vi "leybold QMH.vi"() -> ()   [LabVIEW 2023]
uses:
  usr/local/natinst/LabVIEW-2023-64/examples/Design Patterns/Queued Message Handler/support/QMH Fundamentals - Message Cluster.ctl
  <vilib>/Instr/_visa.llb/VISA Configure Serial Port (Instr).vi
  <vilib>/Utility/error.llb/Error Cluster From Error Code.vi
  <vilib>/ErrorRing/Error Ring.xnode
panel:
  in  "Stop":bool
  in  "recipes":bool
  in  "Tab Control":enum32{"Control", "Vacuum", "Metals", "Oxides"}(tab)
  out "REF Power (W)":i16
  in  "FWD Power (W)":bool=TRUE
  in  "CL":bool
  in  "CT":bool
  in  "RF Source":bool
  out "PFG600":string
  out "read buffer":string
  in  "+100":bool
  out "DC Bias (V)":i16
  in  "Ar (SCCM)":bool
  in  "O2 (SCCM)":bool
  in  "Gas":bool
  in  "+10":bool
  in  "+1":bool
  in  "-1":bool
  in  "-10":bool
  in  "-100":bool
  in  "GAS Boost":bool
  in  "Timer":bool
  in  "Matchbox mode":bool
  in  "TimerOn":bool
  out "PR4000":string
  in  "P1":bool
  in  "P2":bool
  in  "P3":bool
  out "Timer end":timestamp format="%<%H:%M:%S>T"
  out "Time":timestamp format="%<%H:%M:%S\n%x>T"
  in  "RS232":bool
  out "Waveform Chart":waveform(dbl)(graph)
  in  "1h":bool
  in  "8h":bool
  in  "24h":bool
  in  "All":bool
  out "Pressure (mbar)":dbl format="%#_6e"
  # "GENERATOR"
  # "MFC"
  # "TIMER"
  # "PRESETS"
  # "DEBUG"
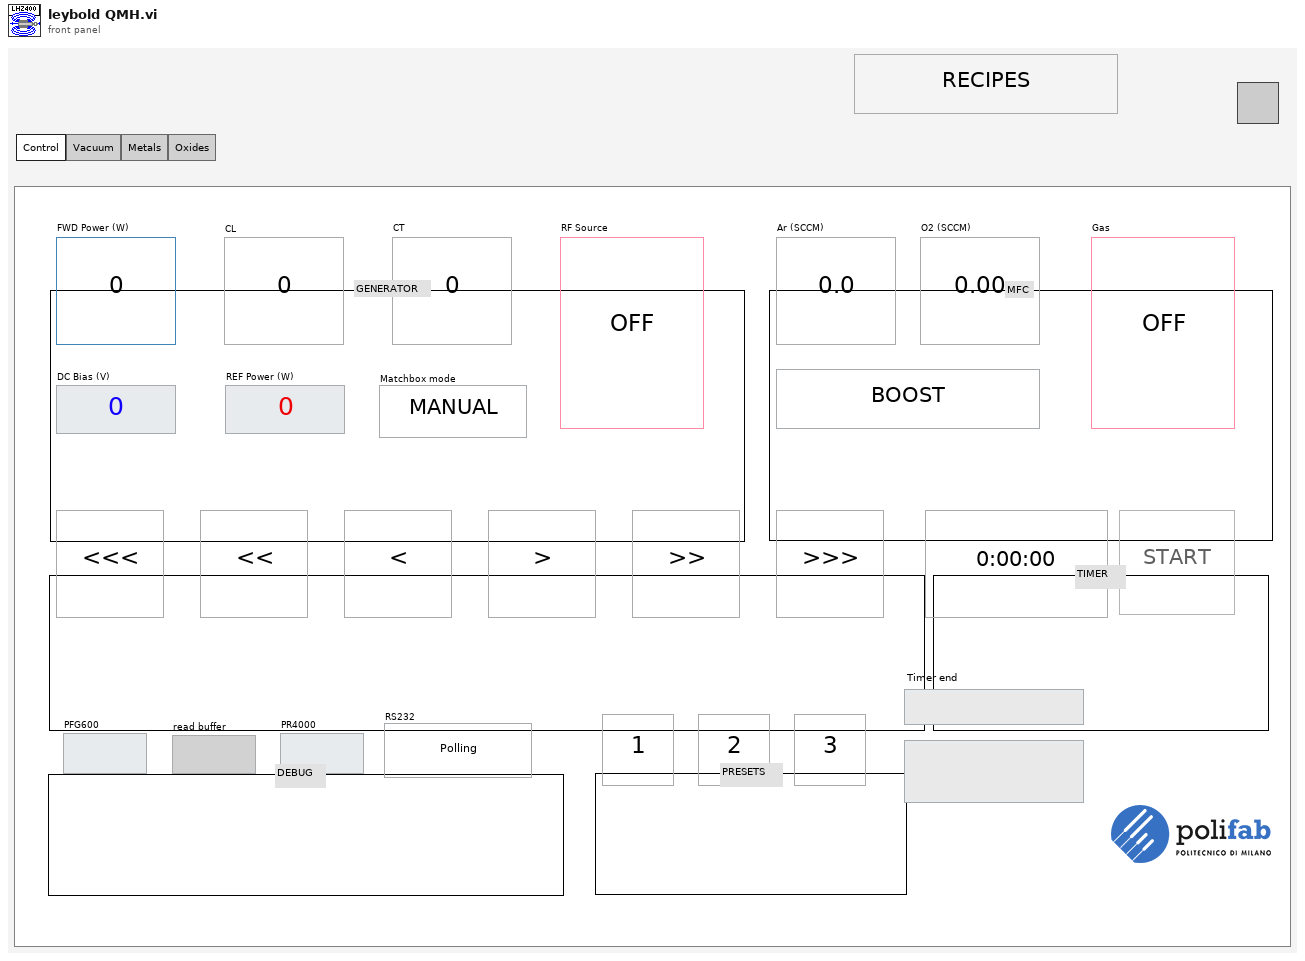
[diagram p1: front panel]
types:
  T1 = typedef "QMH Fundamentals - Message Cluster.ctl" = cluster{"Message":string, "Message Data":variant}
  T2 = cluster{"Message":string, enum16{"FWD", "CL", "CT", "Ar", "O2", "Timer"}}
  T3 = enum8{"Enabled", "Disabled", "Disabled and Grayed Out"}
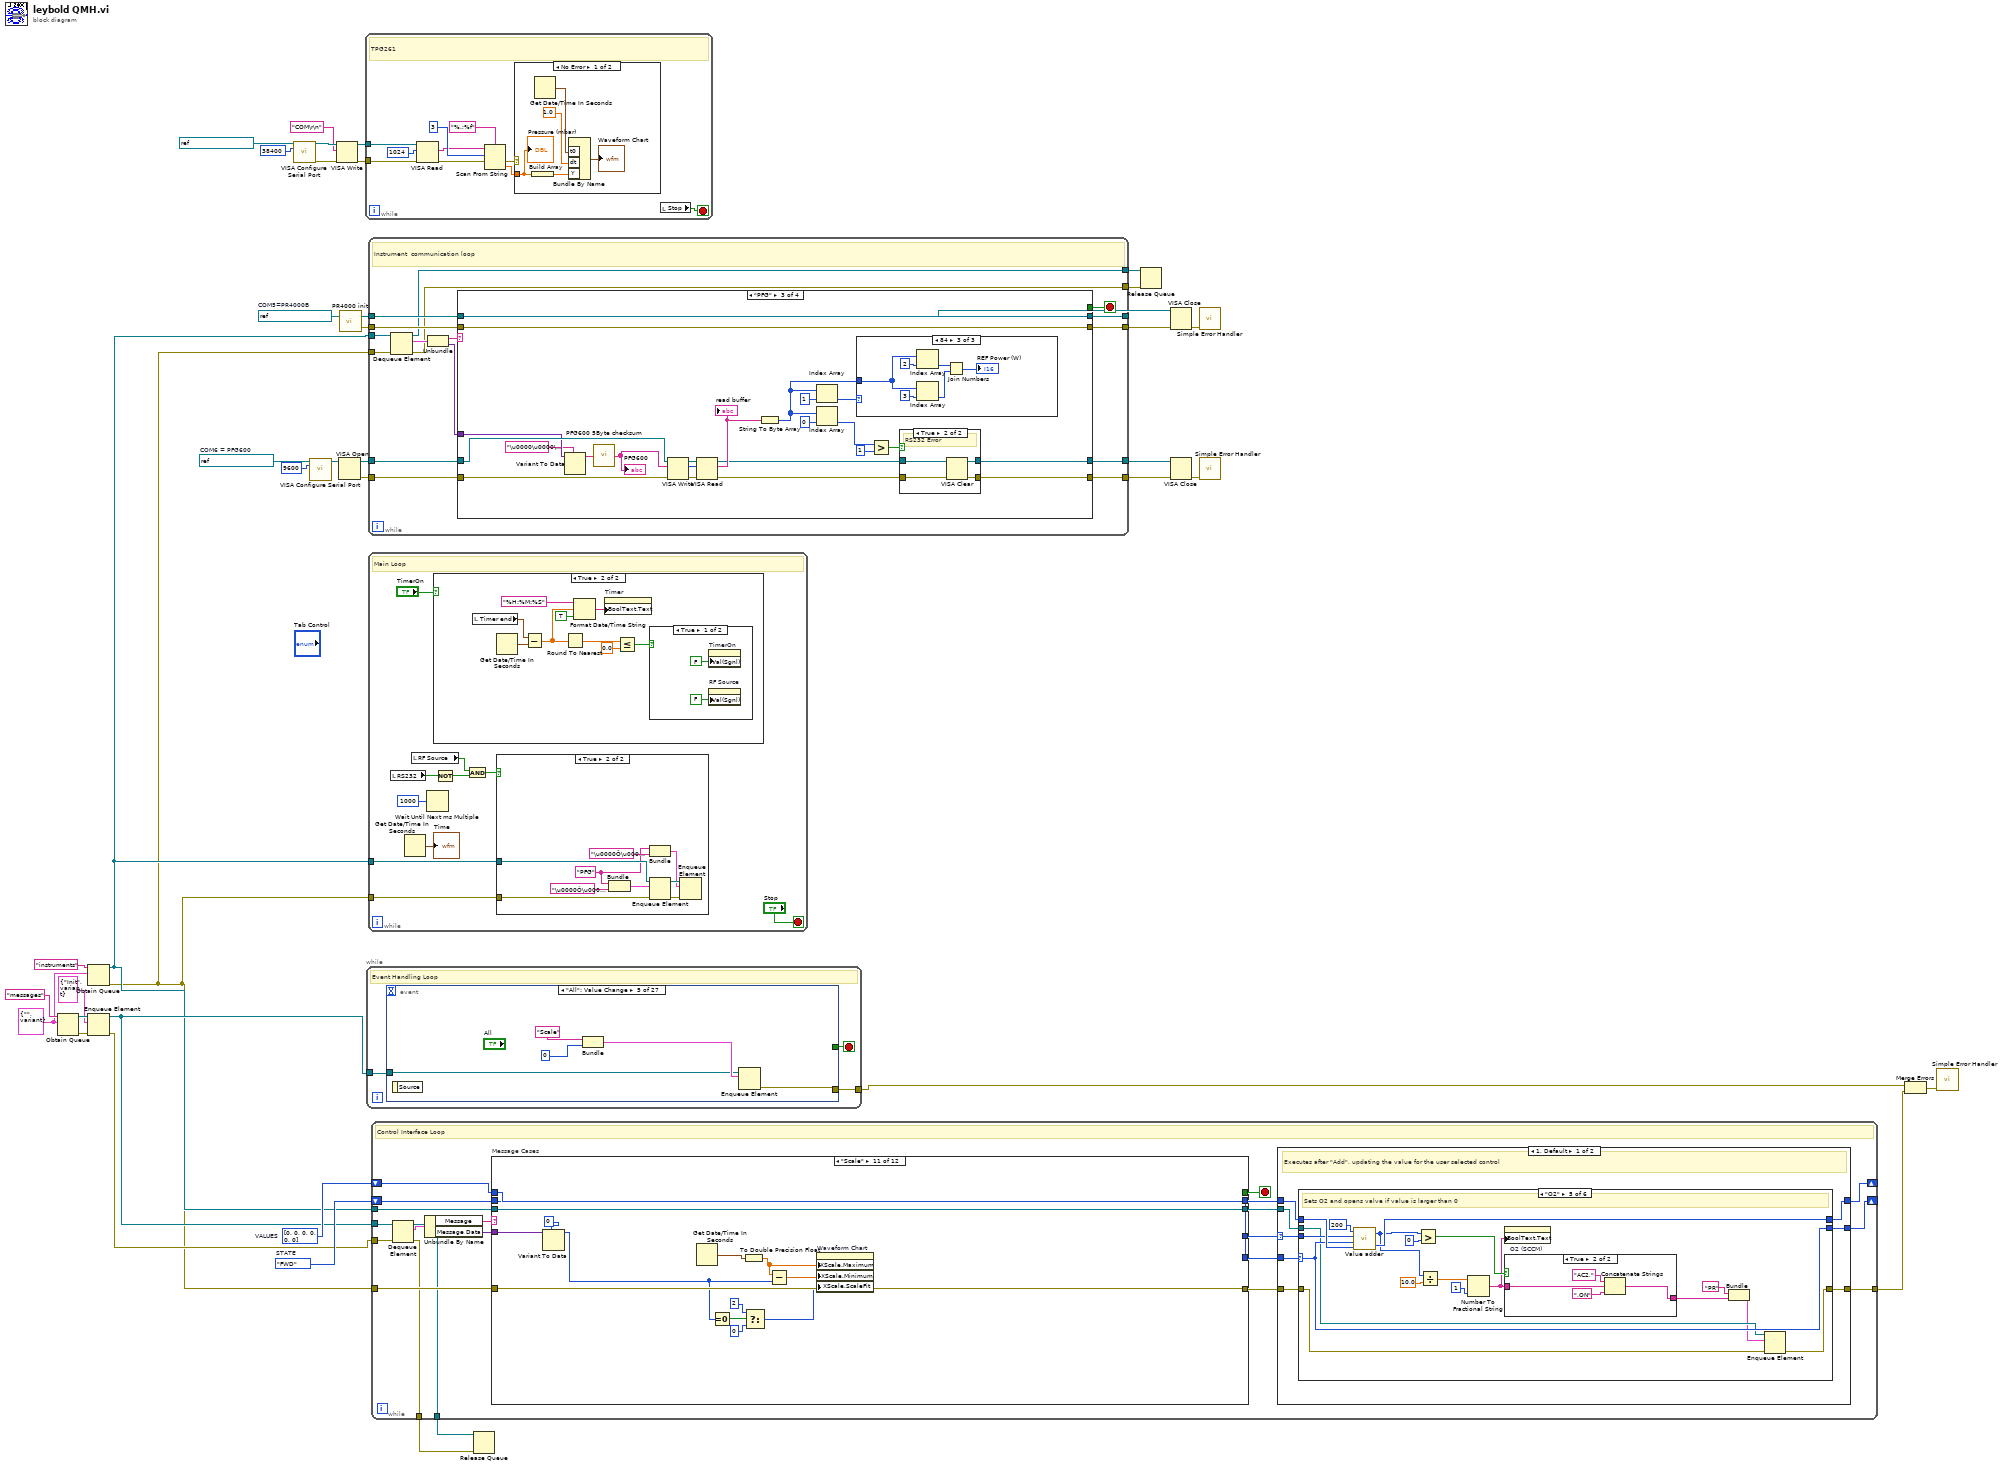
[diagram p0: block diagram]
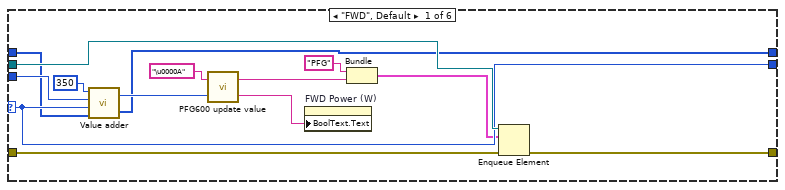
[diagram p2: hidden frame]
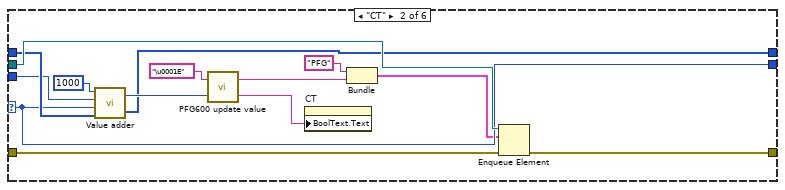
[diagram p3: hidden frame]
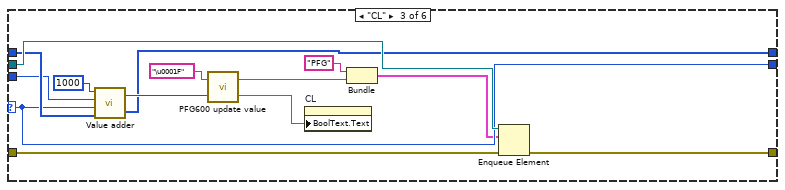
[diagram p4: hidden frame]
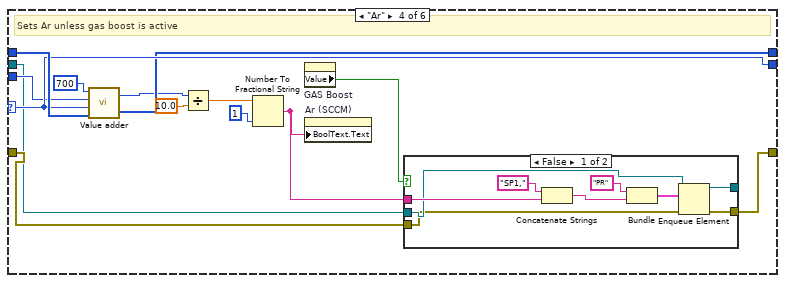
[diagram p5: hidden frame]
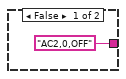
[diagram p7: hidden frame]
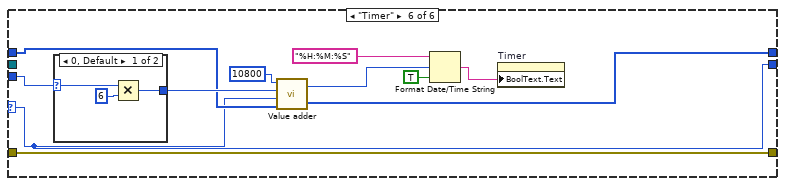
[diagram p8: hidden frame]
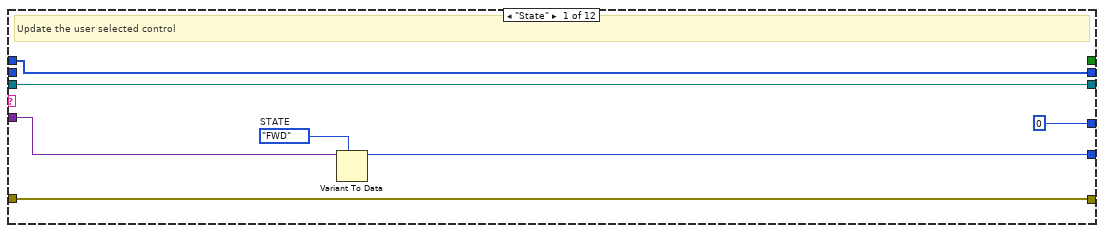
[diagram p11: hidden frame]
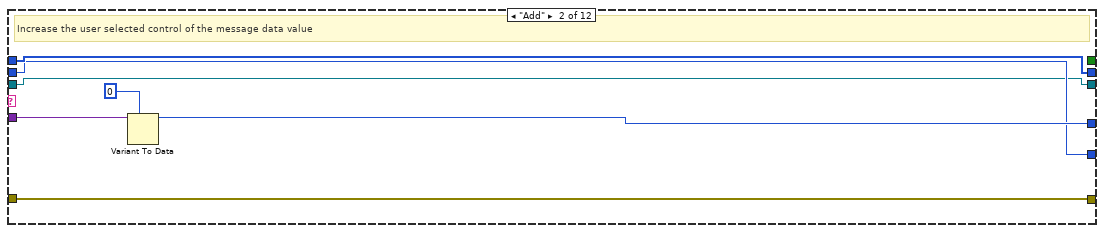
[diagram p12: hidden frame]
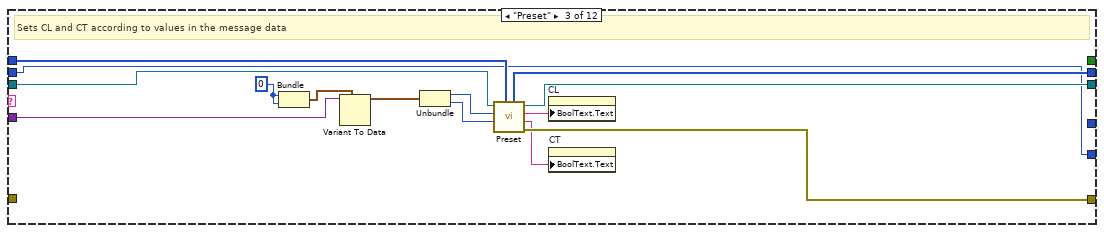
[diagram p13: hidden frame]
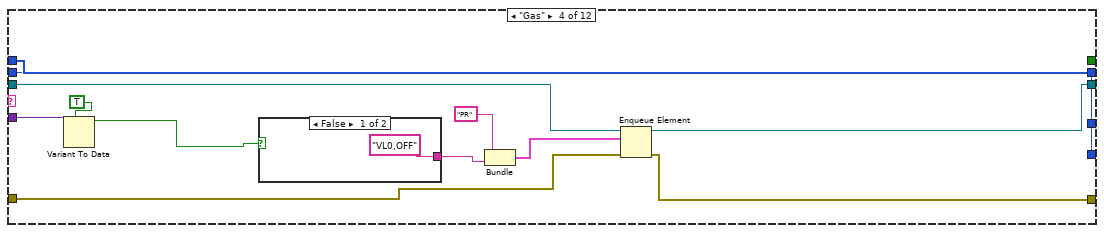
[diagram p14: hidden frame]
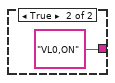
[diagram p15: hidden frame]
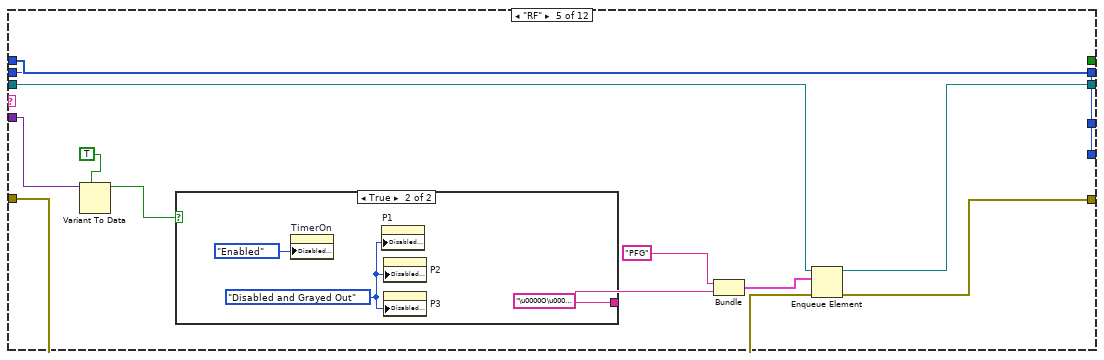
[diagram p16: hidden frame]
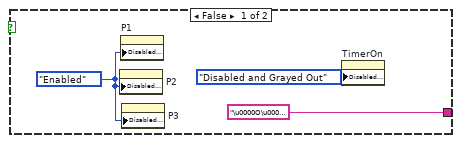
[diagram p17: hidden frame]
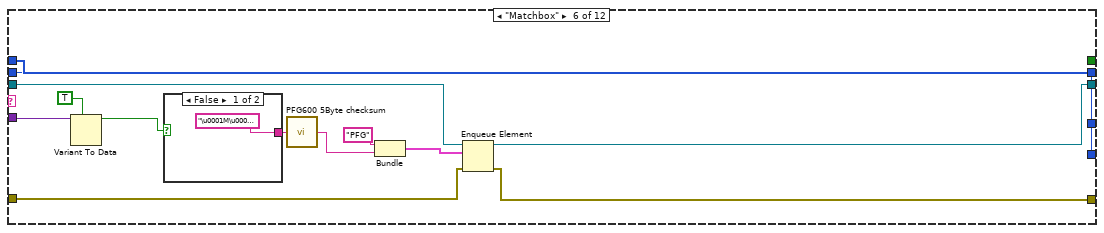
[diagram p18: hidden frame]
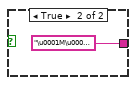
[diagram p19: hidden frame]
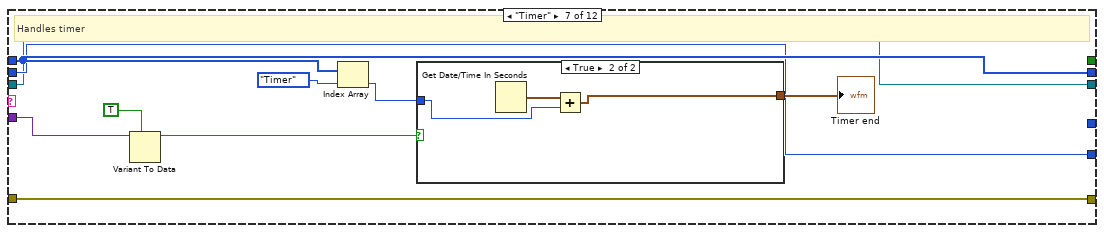
[diagram p20: hidden frame]
diagram:
  w20 = i16[] [0, 0, 0, 0, 0, 0]  # VALUES
  w21 = enum16{"FWD", "CL", "CT", "Ar", "O2", "Timer"}."FWD"  # STATE
  w11 = T1 {"Message"="", "Message Data"=variant} ("Message Cluster")
  w34 = refnum<visa-resource-name> "ASRL33::INSTR"  # COM5=PR4000B
  w5 = refnum<visa-resource-name> "ASRL34::INSTR"  # COM6 = PFG600
  n1 = Obtain Queue(name (unnamed)="messages", element data type=w11) -> (queue out=w25:refnum<queue>, error out=w26:errorcluster)  [unwired: 3 in, 1 out]
  n2 = Obtain Queue(name (unnamed)="instruments", element data type=w11) -> (queue out=w10:refnum<queue>, error out=w9:errorcluster)  [unwired: 3 in, 1 out]
  n3 = Enqueue Element(queue=w25, element=T1 {"Message"="Init", "Message Data"=variant}, error in (no error)=w26) -> (queue out=w19:refnum<queue>, error out=w14:errorcluster)  [unwired: 1 in, 1 out]
  n4 = call-poly "VISA Configure Serial Port"("VISA resource name"=refnum<visa-resource-name> "ASRL36::INSTR", "baud rate (9600)"=u32 38400) -> ("VISA resource name out"=w29:refnum<visa-resource-name>, "error out"=w30:errorcluster)  [unwired: 12 in]
  n5 = call-poly "VISA Configure Serial Port"("VISA resource name"=w5, "baud rate (9600)"=u32 9600) -> ("VISA resource name out"=w6:refnum<visa-resource-name>)  [unwired: 12 in, 1 out]
  n6 = VISA Write(VISA resource name=w29, write buffer="COM\r\n", error in (no error)=w30) -> (VISA resource name out=w31:refnum<visa-resource-name>, error out=w27:errorcluster)  [unwired: 1 out]
  n7 = VISA Open(VISA resource name=w6) -> (VISA resource name=w39:refnum<visa-resource-name>, error out=w40:errorcluster)  [unwired: 4 in]
  n8 = call "PR4000 init.vi"("VISA Refnum in"=w34) -> ("error out"=w17:errorcluster, "VISA Refnum out"=w18:refnum<visa-resource-name>)  [unwired: 1 in]
  n9 = while {
    tunnel: w31 -> [w50]
    tunnel: w27 -> [w49]
    stop <- w41 stop-if-true
    # "TPG261"
    n10 = VISA Read(VISA resource name=w50, byte count=u32 1024, error in (no error)=w49) -> (read buffer=w45:string, error out=w43:errorcluster)  [unwired: 2 out]
    n11 = Scan From String(format string="%.;%f" ("Format-String"), input string=w45, initial scan location=u32 3 ("offset (0)"), error in=w43) -> (error out=w42:errorcluster, output 1=w44:dbl)  [unwired: 1 in, 2 out]
    n12 = case shown="No Error" w42 {
      tunnel: w44 -> [w52 _]
      frame No Error {
        n13 = Build Array(w52) -> (w55:dbl[])
        n14 = Get Date/Time In Seconds() -> (seconds since 1Jan1904=w51:timestamp)
        n15 = Bundle By Name("t0"=w51, "dt"=1.0, "Y"=w55) -> (→"Waveform Chart":waveform(dbl))  [unwired: 1 in]
        "Pressure (mbar)" <- w52
      }
      frame Error {
      }
    }
    n16 = local read "Stop"() -> (w41:bool)
  }
  n17 = while {
    tunnel: w19 -> [w58]
    tunnel: [w56] -> w23
    stop <- w57 stop-if-true
    # "Event Handling Loop"
    n18 = event shown="[4] \"All\": Value Change" {
      selector: _ -> [_ _ _ _ _ _ _ _ _ _ _ _ _ _ _ _ _ _ _ _ _ _ _ _ _ _ _]
      dyn-events: _ -> [_ _ _ _ _ _ _ _ _ _ _ _ _ _ _ _ _ _ _ _ _ _ _ _ _ _ _]
      timeout: _ -> [_ _ _ _ _ _ _ _ _ _ _ _ _ _ _ _ _ _ _ _ _ _ _ _ _ _ _]
      tunnel: [TRUE _ _ _ _ _ _ _ _ _ _ _ _ _ _ _ _ _ _ _ _ _ _ _ _ _ _] -> w57
      tunnel: w58 -> [w62 w64 w69 w74 w79 w83 w89 w93 w97 w101 w105 w109 w112 w115 w118 w121 w124 w129 w134 _ w142 w145 w152 w158 w164 w169 _]
      tunnel: [w61 w63 w68 w73 w78 _ _ _ _ _ _ w108 w111 w114 w117 w120 w123 w128 w133 _ _ _ _ _ _ w168 _] -> w56
      event "Stop": Value Change {
        # "Stop the VI."
        # "Enqueue an \"Exit\" message. Note that the Enqueue Element At Opposite End function is used to place this priority \"Exit\" message at the front of the queue ahead of all other messages."
        n19 = event-data() -> ()  [unwired: 1 in, 1 out]
        n20 = Enqueue Element At Opposite End(queue=w62, element=T1 {"Message"="Exit", "Message Data"=variant}) -> (error out=w61:errorcluster)  [unwired: 2 in, 2 out]
      }
      event "1h": Value Change {
        n21 = event-data() -> ()  [unwired: 1 in, 1 out]
        n22 = Bundle("Scale", 3600) -> (w66:cluster{string, i32})  [unwired: 1 in]
        n23 = Enqueue Element(queue=w64, element=w66) -> (error out=w63:errorcluster)  [unwired: 2 in, 2 out]
      }
      event "8h": Value Change {
        n24 = event-data() -> ()  [unwired: 1 in, 1 out]
        n25 = Bundle("Scale", 28800) -> (w71:cluster{string, i32})  [unwired: 1 in]
        n26 = Enqueue Element(queue=w69, element=w71) -> (error out=w68:errorcluster)  [unwired: 2 in, 2 out]
      }
      event "24h": Value Change {
        n27 = event-data() -> ()  [unwired: 1 in, 1 out]
        n28 = Bundle("Scale", 86400) -> (w76:cluster{string, i32})  [unwired: 1 in]
        n29 = Enqueue Element(queue=w74, element=w76) -> (error out=w73:errorcluster)  [unwired: 2 in, 2 out]
      }
      event "All": Value Change {
        n30 = event-data() -> ()  [unwired: 1 in, 1 out]
        n31 = Bundle("Scale", 0) -> (w81:cluster{string, i32})  [unwired: 1 in]
        n32 = Enqueue Element(queue=w79, element=w81) -> (error out=w78:errorcluster)  [unwired: 2 in, 2 out]
      }
      event "CL": Value Change {
        w86 = FALSE ("FWD Power (W)")
        n33 = event-data() -> ()  [unwired: 1 in, 1 out]
        n34 = Enqueue Element(queue=w83, element=T2 {"Message"="State", enum."CL"}) -> ()  [unwired: 2 in, 3 out]
        n35 = property on="CT" class="Bool (strict)"("Value"=w86) -> ()  [unwired: 2 in, 2 out]
        n36 = property on="Timer" class="Bool (strict)"("Value"=w86) -> ()  [unwired: 2 in, 2 out]
        n37 = property on="CL" class="Bool (strict)"("Value"=TRUE ("CL")) -> ()  [unwired: 2 in, 2 out]
        n38 = property on="Ar (SCCM)" class="Bool (strict)"("Value"=w86) -> ()  [unwired: 2 in, 2 out]
        n39 = property on="O2 (SCCM)" class="Bool (strict)"("Value"=w86) -> ()  [unwired: 2 in, 2 out]
        n40 = property on="FWD Power (W)" class="Bool (strict)"("Value"=w86) -> ()  [unwired: 2 in, 2 out]
      }
      event "CT": Value Change {
        w88 = FALSE ("FWD Power (W)")
        n41 = event-data() -> ()  [unwired: 1 in, 1 out]
        n42 = Enqueue Element(queue=w89, element=T2 {"Message"="State", enum."CT"}) -> ()  [unwired: 2 in, 3 out]
        n43 = property on="CT" class="Bool (strict)"("Value"=TRUE ("CL")) -> ()  [unwired: 2 in, 2 out]
        n44 = property on="CL" class="Bool (strict)"("Value"=w88) -> ()  [unwired: 2 in, 2 out]
        n45 = property on="Timer" class="Bool (strict)"("Value"=w88) -> ()  [unwired: 2 in, 2 out]
        n46 = property on="Ar (SCCM)" class="Bool (strict)"("Value"=w88) -> ()  [unwired: 2 in, 2 out]
        n47 = property on="O2 (SCCM)" class="Bool (strict)"("Value"=w88) -> ()  [unwired: 2 in, 2 out]
        n48 = property on="FWD Power (W)" class="Bool (strict)"("Value"=w88) -> ()  [unwired: 2 in, 2 out]
      }
      event "Ar (SCCM)": Value Change {
        w92 = FALSE ("FWD Power (W)")
        n49 = event-data() -> ()  [unwired: 1 in, 1 out]
        n50 = Enqueue Element(queue=w93, element=T2 {"Message"="State", enum."Ar"}) -> ()  [unwired: 2 in, 3 out]
        n51 = property on="CL" class="Bool (strict)"("Value"=w92) -> ()  [unwired: 2 in, 2 out]
        n52 = property on="Ar (SCCM)" class="Bool (strict)"("Value"=TRUE ("CL")) -> ()  [unwired: 2 in, 2 out]
        n53 = property on="Timer" class="Bool (strict)"("Value"=w92) -> ()  [unwired: 2 in, 2 out]
        n54 = property on="CT" class="Bool (strict)"("Value"=w92) -> ()  [unwired: 2 in, 2 out]
        n55 = property on="O2 (SCCM)" class="Bool (strict)"("Value"=w92) -> ()  [unwired: 2 in, 2 out]
        n56 = property on="FWD Power (W)" class="Bool (strict)"("Value"=w92) -> ()  [unwired: 2 in, 2 out]
      }
      event "O2 (SCCM)": Value Change {
        w96 = FALSE ("FWD Power (W)")
        n57 = event-data() -> ()  [unwired: 1 in, 1 out]
        n58 = Enqueue Element(queue=w97, element=T2 {"Message"="State", enum."O2"}) -> ()  [unwired: 2 in, 3 out]
        n59 = property on="CL" class="Bool (strict)"("Value"=w96) -> ()  [unwired: 2 in, 2 out]
        n60 = property on="O2 (SCCM)" class="Bool (strict)"("Value"=TRUE ("CL")) -> ()  [unwired: 2 in, 2 out]
        n61 = property on="Timer" class="Bool (strict)"("Value"=w96) -> ()  [unwired: 2 in, 2 out]
        n62 = property on="CT" class="Bool (strict)"("Value"=w96) -> ()  [unwired: 2 in, 2 out]
        n63 = property on="Ar (SCCM)" class="Bool (strict)"("Value"=w96) -> ()  [unwired: 2 in, 2 out]
        n64 = property on="FWD Power (W)" class="Bool (strict)"("Value"=w96) -> ()  [unwired: 2 in, 2 out]
      }
      event "FWD Power (W)": Value Change {
        w100 = FALSE ("FWD Power (W)")
        n65 = event-data() -> ()  [unwired: 1 in, 1 out]
        n66 = Enqueue Element(queue=w101, element=T2 {"Message"="State", enum."FWD"}) -> ()  [unwired: 2 in, 3 out]
        n67 = property on="FWD Power (W)" class="Bool (strict)"("Value"=TRUE ("CL")) -> ()  [unwired: 2 in, 2 out]
        n68 = property on="O2 (SCCM)" class="Bool (strict)"("Value"=w100) -> ()  [unwired: 2 in, 2 out]
        n69 = property on="Timer" class="Bool (strict)"("Value"=w100) -> ()  [unwired: 2 in, 2 out]
        n70 = property on="CL" class="Bool (strict)"("Value"=w100) -> ()  [unwired: 2 in, 2 out]
        n71 = property on="Ar (SCCM)" class="Bool (strict)"("Value"=w100) -> ()  [unwired: 2 in, 2 out]
        n72 = property on="CT" class="Bool (strict)"("Value"=w100) -> ()  [unwired: 2 in, 2 out]
      }
      event "Timer": Value Change {
        w103 = FALSE ("FWD Power (W)")
        n73 = event-data() -> ()  [unwired: 1 in, 1 out]
        n74 = Enqueue Element(queue=w105, element=T2 {"Message"="State", enum."Timer"}) -> ()  [unwired: 2 in, 3 out]
        n75 = property on="CT" class="Bool (strict)"("Value"=w103) -> ()  [unwired: 2 in, 2 out]
        n76 = property on="Timer" class="Bool (strict)"("Value"=TRUE ("CL")) -> ()  [unwired: 2 in, 2 out]
        n77 = property on="CL" class="Bool (strict)"("Value"=w103) -> ()  [unwired: 2 in, 2 out]
        n78 = property on="Ar (SCCM)" class="Bool (strict)"("Value"=w103) -> ()  [unwired: 2 in, 2 out]
        n79 = property on="O2 (SCCM)" class="Bool (strict)"("Value"=w103) -> ()  [unwired: 2 in, 2 out]
        n80 = property on="FWD Power (W)" class="Bool (strict)"("Value"=w103) -> ()  [unwired: 2 in, 2 out]
      }
      event "-100": Value Change {
        n81 = event-data() -> ()  [unwired: 1 in, 1 out]
        n82 = Enqueue Element(queue=w109, element=cluster{"Message":string, i32} {"Message"="Add", -100}) -> (error out=w108:errorcluster)  [unwired: 2 in, 2 out]
      }
      event "-10": Value Change {
        n83 = event-data() -> ()  [unwired: 1 in, 1 out]
        n84 = Enqueue Element(queue=w112, element=cluster{"Message":string, i32} {"Message"="Add", -10}) -> (error out=w111:errorcluster)  [unwired: 2 in, 2 out]
      }
      event "-1": Value Change {
        n85 = event-data() -> ()  [unwired: 1 in, 1 out]
        n86 = Enqueue Element(queue=w115, element=cluster{"Message":string, i32} {"Message"="Add", -1}) -> (error out=w114:errorcluster)  [unwired: 2 in, 2 out]
      }
      event "+1": Value Change {
        n87 = event-data() -> ()  [unwired: 1 in, 1 out]
        n88 = Enqueue Element(queue=w118, element=cluster{"Message":string, i32} {"Message"="Add", 1}) -> (error out=w117:errorcluster)  [unwired: 2 in, 2 out]
      }
      event "+10": Value Change {
        n89 = event-data() -> ()  [unwired: 1 in, 1 out]
        n90 = Enqueue Element(queue=w121, element=cluster{"Message":string, i32} {"Message"="Add", 10}) -> (error out=w120:errorcluster)  [unwired: 2 in, 2 out]
      }
      event "+100": Value Change {
        n91 = event-data() -> ()  [unwired: 1 in, 1 out]
        n92 = Enqueue Element(queue=w124, element=cluster{"Message":string, i32} {"Message"="Add", 100}) -> (error out=w123:errorcluster)  [unwired: 2 in, 2 out]
      }
      event "GAS Boost": Value Change {
        n93 = event-data() -> ()  [unwired: 1 in, 1 out]
        n94 = Bundle("Message"="Boost", "GAS Boost"="GAS Boost") -> (w125:cluster{"Message":string, "GAS Boost":bool})  [unwired: 1 in]
        n95 = Enqueue Element(queue=w129, element=w125) -> (error out=w128:errorcluster)  [unwired: 2 in, 2 out]
      }
      event "Gas": Value Change {
        n96 = event-data() -> ()  [unwired: 1 in, 1 out]
        n97 = Bundle("Gas", "Gas"="Gas") -> (w132:cluster{string, "Gas":bool})  [unwired: 1 in]
        n98 = Enqueue Element(queue=w134, element=w132) -> (error out=w133:errorcluster)  [unwired: 2 in, 2 out]
      }
      event "RS232": Value Change {
        n99 = event-data() -> ()  [unwired: 1 in, 1 out]
        n100 = case shown="True" "RS232" {
          tunnel: [T3."Enabled" ("Disabled") T3."Disabled and Grayed Out" ("Disabled")] -> w135
          frame False {
          }
          frame True {
          }
        }
        n101 = property on="DC Bias (V)" class="DigNum (strict)"("DisabledEnum"=w135) -> ()  [unwired: 2 in, 2 out]
        n102 = property on="REF Power (W)" class="DigNum (strict)"("DisabledEnum"=w135) -> ()  [unwired: 2 in, 2 out]
      }
      event "TimerOn": Value Change {
        n103 = event-data() -> ("NewVal"=w141:bool)  [unwired: 1 in]
        n104 = Bundle("Timer", "NewVal"=w141) -> (w139:cluster{string, "NewVal":bool})  [unwired: 1 in]
        n105 = Enqueue Element(queue=w142, element=w139) -> ()  [unwired: 2 in, 3 out]
      }
      event "RF Source": Value Change {
        n106 = event-data() -> ()  [unwired: 1 in, 1 out]
        n107 = Bundle("RF", "RF Source"="RF Source") -> (w144:cluster{string, "RF Source":bool})  [unwired: 1 in]
        n108 = Enqueue Element(queue=w145, element=w144) -> ()  [unwired: 2 in, 3 out]
      }
      event "P1": Value Change {
        n109 = event-data() -> ()  [unwired: 1 in, 1 out]
        n110 = Bundle(0, 1000) -> (w149:cluster{i32, i32})  [unwired: 1 in]
        n111 = Bundle("Preset", w149) -> (w150:cluster{string, cluster{i32, i32}})  [unwired: 1 in]
        n112 = Enqueue Element(queue=w152, element=w150) -> ()  [unwired: 2 in, 3 out]
      }
      event "P2": Value Change {
        n113 = event-data() -> ()  [unwired: 1 in, 1 out]
        n114 = Bundle(250, 750) -> (w155:cluster{i32, i32})  [unwired: 1 in]
        n115 = Bundle("Preset", w155) -> (w156:cluster{string, cluster{i32, i32}})  [unwired: 1 in]
        n116 = Enqueue Element(queue=w158, element=w156) -> ()  [unwired: 2 in, 3 out]
      }
      event "P3": Value Change {
        n117 = event-data() -> ()  [unwired: 1 in, 1 out]
        n118 = Bundle(680, 580) -> (w161:cluster{i32, i32})  [unwired: 1 in]
        n119 = Bundle("Preset", w161) -> (w162:cluster{string, cluster{i32, i32}})  [unwired: 1 in]
        n120 = Enqueue Element(queue=w164, element=w162) -> ()  [unwired: 2 in, 3 out]
      }
      event "Matchbox mode": Value Change {
        n121 = event-data() -> ()  [unwired: 1 in, 1 out]
        n122 = Bundle("Matchbox", "Matchbox mode"="Matchbox mode") -> (w165:cluster{string, "Matchbox mode":bool})  [unwired: 1 in]
        n123 = Enqueue Element(queue=w169, element=w165) -> (error out=w168:errorcluster)  [unwired: 2 in, 2 out]
      }
      event "recipes": Value Change {
        n124 = event-data() -> ()  [unwired: 1 in, 1 out]
        n125 = call <vilib>:"System Exec.vi"("wait until completion? (T)"=FALSE, "command line"="firefox https://docs.google.com/spreadsheets/d/1f53240c20IwFszMSA94HhWp93EeL4Y7tCwhda4_pTaQ/edit#gid=1759381600 ") -> ()  [unwired: 6 in, 4 out]
      }
    }
  }
  n126 = while {
    tunnel: w10 -> [w173]
    tunnel: w9 -> [w172]
    stop <- "Stop" stop-if-true
    # "Main Loop"
    n127 = local read "RS232"() -> (w175:bool)
    n128 = Get Date/Time In Seconds() -> (seconds since 1Jan1904=→"Time":timestamp)
    n129 = local read "RF Source"() -> (w177:bool)
    n130 = Wait Until Next ms Multiple(millisecond multiple=u32 1000 ("milliseconds to wait")) -> ()  [unwired: 1 out]
    n131 = case shown="True" "TimerOn" {
      frame False {
      }
      frame True {
        n132 = local read "Timer end"() -> (w199:timestamp)
        n133 = Get Date/Time In Seconds() -> (seconds since 1Jan1904=w198:timestamp)
        n134 = Subtract(x=w199, y=w198) -> (x-y=w191:dbl)
        n135 = Round To Nearest(number=w191) -> (nearest integer value=w197:dbl)
        n136 = Format Date/Time String(time format string (%c)="%H:%M:%S", seconds (now)=w191, UTC format=TRUE) -> (date/time string=w192:string)
        n137 = property on="Timer" class="Bool (strict)"("BoolText.Text"=w192) -> ()  [unwired: 2 in, 2 out]
        n138 = Less Or Equal?(x=w197, y=0.0) -> (x <= y?=w195:bool)
        n139 = case shown="True" w195 {
          frame True {
            n140 = property on="TimerOn" class="Bool (strict)"("Val(Sgnl)"=FALSE ("Value (Signaling)")) -> ()  [unwired: 2 in, 2 out]
            n141 = property on="RF Source" class="Bool (strict)"("Val(Sgnl)"=FALSE ("RF Source")) -> ()  [unwired: 2 in, 2 out]
          }
          frame False {
          }
        }
      }
    }
    n142 = Not(x=w175) -> (.not. x?=w176:bool)
    n143 = And(x=w177, y=w176) -> (x .and. y?=w178:bool)
    n144 = case shown="True" w178 {
      tunnel: w173 -> [_ w187]
      tunnel: w172 -> [_ w182]
      frame False {
      }
      frame True {
        w184 = "PFG"
        n145 = Bundle(w184, "Input"="\u0000Ò\u0000\u0000") -> (w186:cluster{string, "Input":string})  [unwired: 1 in]
        n146 = Bundle(w184, "Input"="\u0000Ô\u0000\u0000") -> (w183:cluster{string, "Input":string})  [unwired: 1 in]
        n147 = Enqueue Element(queue=w187, element=w186, error in (no error)=w182) -> (queue out=w190:refnum<queue>, error out=w189:errorcluster)  [unwired: 1 in, 1 out]
        n148 = Enqueue Element(queue=w190, element=w183, error in (no error)=w189) -> ()  [unwired: 1 in, 3 out]
      }
    }
  }
  n149 = while {
    tunnel: w9 -> [w206]
    tunnel: w10 -> [w207]
    tunnel: w40 -> [w217]
    tunnel: w39 -> [w216]
    tunnel: [w214] -> w38
    tunnel: [w215] -> w37
    tunnel: w18 -> [w212]
    tunnel: w17 -> [w211]
    tunnel: [w210] -> w16
    tunnel: [w209] -> w15
    tunnel: [w204] -> w1
    tunnel: [w203] -> w2
    stop <- w202 stop-if-true
    # "Instrument  communication loop"
    n150 = Dequeue Element(queue=w207, error in (no error)=w206) -> (queue out=w204:refnum<queue>, element=w205:T1, error out=w203:errorcluster)  [unwired: 1 in, 1 out]
    n151 = Unbundle(w205) -> ("Message"=w213:string, "Message Data"=w208:variant)
    n152 = case shown="\"PFG\"" w213 {
      tunnel: w217 -> [w221 w225 w247 w272]
      tunnel: w216 -> [w220 w224 w246 w273]
      tunnel: [w220 w224 w235 w273] -> w215
      tunnel: [w221 w225 w234 w272] -> w214
      tunnel: w212 -> [w219 w222 w231 w276]
      tunnel: w211 -> [w218 w223 w232 w275]
      tunnel: [w218 w223 w232 w274] -> w210
      tunnel: [w219 w222 w231 w271] -> w209
      tunnel: w208 -> [_ _ w230 w269]
      tunnel: [_ TRUE _ _] -> w202
      frame Default {
      }
      frame "Exit" {
      }
      frame "PFG" {
        n153 = Variant To Data(type="\u0000\u0000\u0000\u0000", Variant=w230) -> (data=w228:string)  [unwired: 1 in, 1 out]
        n154 = call "PFG600 5Byte checksum.vi"("Input"=w228) -> ("Output"=w227:string)
        "PFG600" <- w227
        n155 = VISA Write(VISA resource name=w246, write buffer=w227, error in (no error)=w247) -> (VISA resource name out=w249:refnum<visa-resource-name>, return count=w242:u32, error out=w248:errorcluster)
        n156 = VISA Read(VISA resource name=w249, byte count=w242, error in (no error)=w248) -> (VISA resource name out=w236:refnum<visa-resource-name>, read buffer=w245:string, error out=w233:errorcluster)  [unwired: 1 out]
        "read buffer" <- w245
        n157 = String To Byte Array(string=w245) -> (unsigned byte array=w241:u8[])
        n158 = Index Array(array=w241, index=1) -> (element=w243:u8)
        n159 = Index Array(array=w241, index=0) -> (element=w239:u8)
        n160 = case shown="84" w243 {
          tunnel: w241 -> [_ w257 w263]
          frame Default {
          }
          frame 82 {
            n161 = Index Array(array=w257, index=2) -> (element=w261:u8)
            n162 = Index Array(array=w257, index=3) -> (element=w259:u8)
            n163 = Join Numbers(hi=w261, lo=w259) -> ((hi.lo)=→"DC Bias (V)":u16)
          }
          frame 84 {
            n164 = Index Array(array=w263, index=2) -> (element=w267:u8)
            n165 = Index Array(array=w263, index=3) -> (element=w265:u8)
            n166 = Join Numbers(hi=w267, lo=w265) -> ((hi.lo)=→"REF Power (W)":u16)
          }
        }
        n167 = Greater?(x=w239, y=u8 1) -> (0:w237:bool)
        n168 = case shown="True" w237 {
          tunnel: w236 -> [w251 w255]
          tunnel: w233 -> [w250 w254]
          tunnel: [w250 w253] -> w234
          tunnel: [w251 w252] -> w235
          frame False {
          }
          frame True {
            # "RS232 Error"
            n169 = VISA Clear(VISA resource name=w255, error in (no error)=w254) -> (VISA resource name out=w252:refnum<visa-resource-name>, error out=w253:errorcluster)
          }
        }
      }
      frame "PR" {
        n170 = Variant To Data(type="", Variant=w269) -> (data=w268:string)  [unwired: 1 in, 1 out]
        "PR4000" <- w268
        n171 = VISA Write(VISA resource name=w276, write buffer=w268, error in (no error)=w275) -> (VISA resource name out=w271:refnum<visa-resource-name>, error out=w274:errorcluster)  [unwired: 1 out]
      }
    }
  }
  n172 = while {
    tunnel: w19 -> [w293]
    tunnel: w14 -> [w292]
    shift-right: [w289] -> _
    shift-left: w20 -> [w288]
    shift-right: [w283] -> _
    shift-left: w21 -> [w291]
    tunnel: w10 -> [w282]
    tunnel: [w280] -> w8
    tunnel: w9 -> [w279]
    tunnel: [w278] -> w4
    tunnel: [w277] -> w3
    stop <- w281 stop-if-true
    # "Control Interface Loop"
    n173 = Dequeue Element(queue=w293, error in (no error)=w292) -> (queue out=w278:refnum<queue>, element=w296:T1, error out=w277:errorcluster)  [unwired: 1 in, 1 out]
    n174 = Unbundle By Name(w296) -> ("Message"=w295:string, "Message Data"=w294:variant)
    n175 = case "Message Cases" shown="\"Scale\"" w295 {
      selector: w295 -> [_ _ _ _ _ _ _ _ _ w540 _ w562]
      tunnel: w294 -> [w419 w426 w440 w447 w458 w475 w493 w516 _ w539 w554 _]
      tunnel: [w416 w423 w431 w452 w466 w485 w491 w514 w536 w546 w560 w566] -> w285
      tunnel: w291 -> [_ w422 w428 w451 w465 w484 w490 w507 w535 w545 w557 w565]
      tunnel: [0 w424 _ _ _ _ _ 0 _ _ _ 0] -> w290
      tunnel: w288 -> [w416 w423 w432 w452 w466 w485 w491 w514 w536 w546 w560 w566]
      tunnel: [w414 w421 w434 w442 w459 w479 w489 w510 w534 w543 w559 w564] -> w287
      tunnel: [w413 w420 w433 w449 w460 w478 w488 w509 w528 w537 w558 w561] -> w286
      tunnel: [w415 w422 w428 w451 w465 w484 w490 w507 w535 w545 w557 w565] -> w284
      tunnel: w282 -> [w414 w421 w427 w450 w461 w480 w489 w506 w534 w542 w559 w564]
      tunnel: [_ _ _ _ _ _ _ _ _ TRUE _ _] -> w281
      tunnel: w279 -> [w413 w420 _ w441 w455 w473 w488 _ w528 w538 w558 w561]
      frame "State" {
        w417 = enum16{"FWD", "CL", "CT", "Ar", "O2", "Timer"}."FWD"  # STATE
        # "Update the user selected control"
        n176 = Variant To Data(type=w417, Variant=w419) -> (data=w415:enum16{"FWD", "CL", "CT", "Ar", "O2", "Timer"})  [unwired: 1 in, 1 out]
      }
      frame "Add" {
        # "Increase the user selected control of the message data value"
        n177 = Variant To Data(type=0, Variant=w426) -> (data=w424:i32)  [unwired: 1 in, 1 out]
      }
      frame "Preset" {
        w439 = 0
        # "Sets CL and CT according to values in the message data"
        n178 = Bundle(w439, w439) -> (w438:cluster{i32, i32})  [unwired: 1 in]
        n179 = Variant To Data(type=w438, Variant=w440) -> (data=w437:cluster{i32, i32})  [unwired: 1 in, 1 out]
        n180 = Unbundle(w437) -> (w436:i32, w435:i32)
        n181 = call "Preset.vi"("Array"=w432, "CT"=w435, "CL"=w436, "queue in"=w427) -> ("error out"=w433:errorcluster, "Text CT"=w429:string, "Text CL"=w430:string, "queue out"=w434:refnum<queue>, "output array"=w431:i16[])  [unwired: 3 in]
        n182 = property on="CL" class="Bool (strict)"("BoolText.Text"=w430) -> ()  [unwired: 2 in, 2 out]
        n183 = property on="CT" class="Bool (strict)"("BoolText.Text"=w429) -> ()  [unwired: 2 in, 2 out]
      }
      frame "Gas" {
        n184 = Variant To Data(type=TRUE, Variant=w447) -> (data=w445:bool)  [unwired: 1 in, 1 out]
        n185 = case shown="False" w445 {
          tunnel: ["VL0,OFF" ("string") "VL0,ON" ("string")] -> w448
          frame False {
          }
          frame True {
          }
        }
        n186 = Bundle("PR", "string"=w448) -> (w443:cluster{string, "string":string})  [unwired: 1 in]
        n187 = Enqueue Element(queue=w450, element=w443, error in (no error)=w441) -> (queue out=w442:refnum<queue>, error out=w449:errorcluster)  [unwired: 1 in, 1 out]
      }
      frame "RF" {
        n188 = Variant To Data(type=TRUE, Variant=w458) -> (data=w456:bool)  [unwired: 1 in, 1 out]
        n189 = case shown="True" w456 {
          tunnel: ["\u0000O\u0000\u0000" "\u0000O\u0000\u0001"] -> w464
          frame False {
            w467 = T3."Enabled" ("Disabled")
            n190 = property on="P2" class="Bool"("DisabledEnum"=w467) -> ()  [unwired: 2 in, 2 out]
            n191 = property on="P1" class="Bool"("DisabledEnum"=w467) -> ()  [unwired: 2 in, 2 out]
            n192 = property on="P3" class="Bool"("DisabledEnum"=w467) -> ()  [unwired: 2 in, 2 out]
            n193 = property on="TimerOn" class="Bool (strict)"("DisabledEnum"=T3."Disabled and Grayed Out" ("Disabled")) -> ()  [unwired: 2 in, 2 out]
          }
          frame True {
            w470 = T3."Disabled and Grayed Out" ("Disabled")
            n194 = property on="TimerOn" class="Bool (strict)"("DisabledEnum"=T3."Enabled" ("Disabled")) -> ()  [unwired: 2 in, 2 out]
            n195 = property on="P1" class="Bool"("DisabledEnum"=w470) -> ()  [unwired: 2 in, 2 out]
            n196 = property on="P2" class="Bool"("DisabledEnum"=w470) -> ()  [unwired: 2 in, 2 out]
            n197 = property on="P3" class="Bool"("DisabledEnum"=w470) -> ()  [unwired: 2 in, 2 out]
          }
        }
        n198 = Bundle("PFG", w464) -> (w462:cluster{string, string})  [unwired: 1 in]
        n199 = Enqueue Element(queue=w461, element=w462, error in (no error)=w455) -> (queue out=w459:refnum<queue>, error out=w460:errorcluster)  [unwired: 1 in, 1 out]
      }
      frame "Matchbox" {
        n200 = Variant To Data(type=TRUE, Variant=w475) -> (data=w474:bool)  [unwired: 1 in, 1 out]
        n201 = case shown="False" w474 {
          tunnel: ["\u0001M\u0000\u0001" "\u0001M\u0000\u0002"] -> w482
          frame False {
          }
          frame True {
          }
        }
        n202 = call "PFG600 5Byte checksum.vi"("Input"=w482) -> ("Output"=w481:string)
        n203 = Bundle("PFG", "Output"=w481) -> (w477:cluster{string, "Output":string})  [unwired: 1 in]
        n204 = Enqueue Element(queue=w480, element=w477, error in (no error)=w473) -> (queue out=w479:refnum<queue>, error out=w478:errorcluster)  [unwired: 1 in, 1 out]
      }
      frame "Timer" {
        # "Handles timer"
        n205 = Variant To Data(type=TRUE, Variant=w493) -> (data=w492:bool)  [unwired: 1 in, 1 out]
        n206 = Index Array(array=w491, index=enum16{"FWD", "CL", "CT", "Ar", "O2", "Timer"}."Timer") -> (element=w496:i16)
        n207 = case shown="True" w492 {
          tunnel: w496 -> [w498 w503]
          tunnel: [timestamp(0 s since 1904-01-01) w504] -> w497
          frame False {
            n208 = Format Date/Time String(time format string (%c)="%H:%M:%S", seconds (now)=w498, UTC format=TRUE) -> (date/time string=w499:string)
            n209 = property on="Timer" class="Bool (strict)"("BoolText.Text"=w499) -> ()  [unwired: 2 in, 2 out]
          }
          frame True {
            n210 = Get Date/Time In Seconds() -> (seconds since 1Jan1904=w505:timestamp)
            n211 = Add(x=w505, y=w503) -> (x+y=w504:timestamp)
          }
        }
        "Timer end" <- w497
      }
      frame "Boost" {
        # "Sets Ar to 60 SCCM or revert to previous value"
        n212 = Variant To Data(type=TRUE, Variant=w516) -> (data=w508:bool)  [unwired: 1 in, 1 out]
        n213 = case shown="False" w508 {
          tunnel: [w523 "SP1,60.0"] -> w512
          tunnel: w514 -> [w526 _]
          frame False {
            n214 = Index Array(array=w526, index=enum16{"FWD", "CL", "CT", "Ar", "O2", "Timer"}."Ar") -> (element=w520:i16)
            n215 = Divide(x=w520, y=10.0) -> (x/y=w519:dbl)
            n216 = Number To Fractional String(number=w519, precision (6)=i16 1) -> (F-format string=w521:string)  [unwired: 2 in]
            n217 = Concatenate Strings("SP1," ("string"), w521) -> (w523:string)
          }
          frame True {
          }
        }
        n218 = Bundle("PR", w512) -> (w511:cluster{string, string})  [unwired: 1 in]
        n219 = Enqueue Element(queue=w506, element=w511) -> (queue out=w510:refnum<queue>, error out=w509:errorcluster)  [unwired: 2 in, 1 out]
      }
      frame "Init" {
        w529 = "0" ("Boolean Text.Text")
        # "Interface initzialization"
        n220 = property on="Tab Control" class="TabCtl (strict)"("TabHeight"=u32 50 ("Fixed Tab Dimension:Height")) -> ()  [unwired: 2 in, 2 out]
        n221 = property on="CL" class="Bool (strict)"("BoolText.Text"=w529) -> ()  [unwired: 2 in, 2 out]
        n222 = property on="FWD Power (W)" class="Bool (strict)"("BoolText.Text"=w529) -> ()  [unwired: 2 in, 2 out]
        n223 = property on="CT" class="Bool (strict)"("BoolText.Text"=w529) -> ()  [unwired: 2 in, 2 out]
        n224 = property on="Ar (SCCM)" class="Bool (strict)"("BoolText.Text"="0.0") -> ()  [unwired: 2 in, 2 out]
        n225 = invoke class="VI" method="Default Vals.Reinit All"() -> ()  [unwired: 3 in, 3 out]
        n226 = property on="O2 (SCCM)" class="Bool (strict)"("BoolText.Text"="0.00") -> ()  [unwired: 2 in, 2 out]
        n227 = property on="Timer" class="Bool (strict)"("BoolText.Text"="0:00:00" ("Boolean Text.Text")) -> ()  [unwired: 2 in, 2 out]
      }
      frame "Exit" {
        # "Stop the VI."
        # "Releases Queue and exit"
        n228 = Bundle(w540, "Message Data"=w539) -> (w541:cluster{string, "Message Data":variant})  [unwired: 1 in]
        n229 = Enqueue Element(queue=w542, element=w541, error in (no error)=w538) -> (queue out=w543:refnum<queue>, error out=w537:errorcluster)  [unwired: 1 in, 1 out]
      }
      frame "Scale" {
        n230 = Variant To Data(type=0, Variant=w554) -> (data=w550:i32)  [unwired: 1 in, 1 out]
        n231 = Get Date/Time In Seconds() -> (seconds since 1Jan1904=w556:timestamp)
        n232 = Equal To 0?(x=w550) -> (x = 0?=w551:bool)
        n233 = To Double Precision Float(number=w556) -> (double precision float=w555:dbl)
        n234 = Select(t=2, s=w551, f=0) -> (s? t:f=w549:i32)
        n235 = Subtract(x=w555, y=w550) -> (x-y=w552:dbl)
        n236 = property on="Waveform Chart" class="WFChart (strict)"("XScale.Maximum"=w555, "XScale.Minimum"=w552, "XScale.ScaleFit"=w549) -> ()  [unwired: 2 in, 2 out]
      }
      frame Default {
        # "Case not handled"
        n237 = xnode "Error Ring"("parameter 0"=w562) -> ("error out"=w563:errorcluster)
        n238 = call <vilib>:"Simple Error Handler.vi"("error in (no error)"=w563) -> ()  [unwired: 4 in, 5 out]
      }
    }
    n239 = case shown="1, Default" w290 {
      selector: w290 -> [w300 _]
      tunnel: w286 -> [w302 w410]
      tunnel: w285 -> [w304 w412]
      tunnel: [w303 w412] -> w289
      tunnel: w287 -> [w301 _]
      tunnel: w284 -> [w299 w411]
      tunnel: [w298 w411] -> w283
      tunnel: [w297 w410] -> w280
      frame 1, Default {
        # "Executes after \"Add\", updating the value for the user selected control"
        n240 = case shown="\"O2\"" w299 {
          selector: w299 -> [w313 w327 w341 w358 w387 w402]
          tunnel: [w313 w327 w341 w358 w387 w402] -> w298
          tunnel: w304 -> [w312 w328 w342 w359 w388 w403]
          tunnel: w300 -> [w314 w326 w340 w357 w386 w400]
          tunnel: [w310 w324 w338 w356 w385 w401] -> w303
          tunnel: w301 -> [w317 w331 w345 w348 w377 _]
          tunnel: w302 -> [w316 w330 w344 w351 w378 w395]
          tunnel: [w305 w319 w333 w347 w372 w395] -> w297
          frame "FWD", Default {
            n241 = call "Value adder.vi"("Array"=w312, "Enum"=w313, "value"=w314, "Max Limit"=i16 350) -> ("output array"=w310:i16[], "Limited value"=w311:i16)
            n242 = call "PFG600 update value.vi"("Value"=w311, "Command"="\u0000A") -> ("Text"=w309:string, "Hex"=w308:string)
            n243 = property on="FWD Power (W)" class="Bool (strict)"("BoolText.Text"=w309) -> ()  [unwired: 2 in, 2 out]
            n244 = Bundle("PFG", "Hex"=w308) -> (w306:cluster{string, "Hex":string})  [unwired: 1 in]
            n245 = Enqueue Element(queue=w317, element=w306, error in (no error)=w316) -> (error out=w305:errorcluster)  [unwired: 1 in, 2 out]
          }
          frame "CT" {
            n246 = call "Value adder.vi"("Array"=w328, "Enum"=w327, "value"=w326, "Max Limit"=i16 1000) -> ("output array"=w324:i16[], "Limited value"=w325:i16)
            n247 = call "PFG600 update value.vi"("Value"=w325, "Command"="\u0001E") -> ("Text"=w323:string, "Hex"=w321:string)
            n248 = property on="CT" class="Bool (strict)"("BoolText.Text"=w323) -> ()  [unwired: 2 in, 2 out]
            n249 = Bundle("PFG", "Hex"=w321) -> (w320:cluster{string, "Hex":string})  [unwired: 1 in]
            n250 = Enqueue Element(queue=w331, element=w320, error in (no error)=w330) -> (error out=w319:errorcluster)  [unwired: 1 in, 2 out]
          }
          frame "CL" {
            n251 = call "Value adder.vi"("Array"=w342, "Enum"=w341, "value"=w340, "Max Limit"=i16 1000) -> ("output array"=w338:i16[], "Limited value"=w339:i16)
            n252 = call "PFG600 update value.vi"("Value"=w339, "Command"="\u0001F") -> ("Text"=w334:string, "Hex"=w336:string)
            n253 = property on="CL" class="Bool (strict)"("BoolText.Text"=w334) -> ()  [unwired: 2 in, 2 out]
            n254 = Bundle("PFG", "Hex"=w336) -> (w335:cluster{string, "Hex":string})  [unwired: 1 in]
            n255 = Enqueue Element(queue=w345, element=w335, error in (no error)=w344) -> (error out=w333:errorcluster)  [unwired: 1 in, 2 out]
          }
          frame "Ar" {
            # "Sets Ar unless gas boost is active"
            n256 = call "Value adder.vi"("Array"=w359, "Enum"=w358, "value"=w357, "Max Limit"=i16 700) -> ("output array"=w356:i16[], "Limited value"=w354:i16)
            n257 = Divide(x=w354, y=10.0) -> (x/y=w353:dbl)
            n258 = Number To Fractional String(number=w353, precision (6)=i16 1) -> (F-format string=w350:string)  [unwired: 2 in]
            n259 = property on="GAS Boost" class="Bool (strict)"() -> ("Value"=w349:bool)  [unwired: 2 in, 2 out]
            n260 = property on="Ar (SCCM)" class="Bool (strict)"("BoolText.Text"=w350) -> ()  [unwired: 2 in, 2 out]
            n261 = case shown="False" w349 {
              tunnel: w350 -> [w368 _]
              tunnel: w348 -> [w367 w371]
              tunnel: [w366 w371] -> _
              tunnel: w351 -> [w361 w370]
              tunnel: [w365 w370] -> w347
              frame False {
                n262 = Concatenate Strings("SP1," ("string"), w368) -> (w364:string)
                n263 = Bundle("PR", w364) -> (w362:cluster{string, string})  [unwired: 1 in]
                n264 = Enqueue Element(queue=w367, element=w362, error in (no error)=w361) -> (queue out=w366:refnum<queue>, error out=w365:errorcluster)  [unwired: 1 in, 1 out]
              }
              frame True {
              }
            }
          }
          frame "O2" {
            # "Sets O2 and opens valve if value is larger than 0"
            n265 = call "Value adder.vi"("Array"=w388, "Enum"=w387, "value"=w386, "Max Limit"=i16 200) -> ("output array"=w385:i16[], "Limited value"=w380:i16)
            n266 = Greater?(x=w380, y=i16 0) -> (0:w379:bool)
            n267 = Divide(x=w380, y=10.0) -> (x/y=w383:dbl)
            n268 = Number To Fractional String(number=w383, precision (6)=i16 1) -> (F-format string=w376:string)  [unwired: 2 in]
            n269 = property on="O2 (SCCM)" class="Bool (strict)"("BoolText.Text"=w376) -> ()  [unwired: 2 in, 2 out]
            n270 = case shown="True" w379 {
              tunnel: ["AC2,0,OFF" w391] -> w374
              tunnel: w376 -> [_ w393]
              frame False {
              }
              frame True {
                n271 = Concatenate Strings("AC2," ("string"), w393, ",ON" ("string")) -> (w391:string)
              }
            }
            n272 = Bundle("PR", w374) -> (w373:cluster{string, string})  [unwired: 1 in]
            n273 = Enqueue Element(queue=w377, element=w373, error in (no error)=w378) -> (error out=w372:errorcluster)  [unwired: 1 in, 2 out]
          }
          frame "Timer" {
            n274 = case shown="0, Default" w400 {
              selector: w400 -> [w407 w409]
              tunnel: [w408 w409] -> w404
              frame 0, Default {
                n275 = Multiply(x=w407, y=6) -> (x*y=w408:i32)
              }
              frame -1, 1 {
              }
            }
            n276 = call "Value adder.vi"("Array"=w403, "Enum"=w402, "value"=w404, "Max Limit"=i16 10800) -> ("output array"=w401:i16[], "Limited value"=w399:i16)
            n277 = Format Date/Time String(time format string (%c)="%H:%M:%S", seconds (now)=w399, UTC format=TRUE) -> (date/time string=w396:string)
            n278 = property on="Timer" class="Bool (strict)"("BoolText.Text"=w396) -> ()  [unwired: 2 in, 2 out]
          }
        }
      }
      frame 0 {
        # "Does nothing  for cases different than \"Add\""
      }
    }
  }
  n279 = Release Queue(queue=w4, error in (no error)=w3) -> ()  [unwired: 1 in, 3 out]
  n280 = Release Queue(queue=w1, error in (no error)=w2) -> ()  [unwired: 1 in, 3 out]
  n281 = VISA Close(VISA resource name=w15, error in (no error)=w16) -> (error out=w35:errorcluster)
  n282 = VISA Close(VISA resource name=w37, error in (no error)=w38) -> (error out=w36:errorcluster)
  n283 = call <vilib>:"Simple Error Handler.vi"("error in (no error)"=w35) -> ()  [unwired: 4 in, 5 out]
  n284 = call <vilib>:"Simple Error Handler.vi"("error in (no error)"=w36) -> ()  [unwired: 4 in, 5 out]
  n285 = Merge Errors(w23, w8) -> (w22:errorcluster)
  n286 = call <vilib>:"Simple Error Handler.vi"("error in (no error)"=w22) -> ()  [unwired: 4 in, 5 out]
